vi "Clean Data.vi"(0 "Display State In":T1, 9 "Container State":T3, 11 "error in (no error)":errorcluster) -> (4 "Display State Out":T1, 15 "error out":errorcluster)   [LabVIEW 2017, in "3D Stem.xctl"]
uses:
  <vilib>/Math Plots/3D Math Plots/3D Stem/3D Stem XCtrl/3D Stem.xctl
  <vilib>/_xctls/Container State.ctl
  <vilib>/Math Plots/3D Math Plots/3D Stem/3D Stem XCtrl/State.ctl
  <vilib>/Math Plots/3D Math Plots/3D Stem/3D Stem/3D Stem.lvclass
  <vilib>/Math Plots/3D Math Plots/3D Plot/Action String/3DMathPlot Ctrl Act Queue.ctl
  <vilib>/Math Plots/3D Math Plots/3D Plot/Action String/3DMathPlot Ctrl Act Cluster.ctl
  <vilib>/Math Plots/3D Math Plots/3D Plot/Action String/3DMathPlot State Class.ctl
  <vilib>/_xctls/XControlSupport.lvlib
types:
  T1 = typedef "3D Stem.xctl/State.ctl" = cluster{"3D Stem.lvclass":refnum<class "3D Stem.lvclass">, "Control Ref Queue":T2, "Main Frame Color":u32, "Ramp Palette Color":u32, "Projection Palette Color":u32}
  T2 = typedef "3DMathPlot Ctrl Act Queue.ctl" = refnum<queue>
  T3 = typedef "XControlSupport.lvlib/Container State.ctl" = cluster{"Indicator?":bool, "Run Mode?":bool, " Refnum":refnum<vi>}
  T4 = typedef "3DMathPlot State Class.ctl" = enum16{"Update All Objects (Undo)", "Update Light Object Only", "Update Axis Object Only", "Update Plot Object Only", "Update Cursor Object Only", "Update Axis Plot Cursor Objects", "No Update"}
  T5 = typedef "3DMathPlot Ctrl Act Cluster.ctl" = cluster{"3D Picture Control":refnum<vi>, "Render Window Refnum":refnum<vi>, "XY Graph":refnum<vi>, "Intensity Graph":refnum<vi>, "Color Legend Palette":refnum<vi>, "Projection Palette":refnum<vi>, "XControl  Ref":refnum<vi>, "Facade Ref":refnum<vi>, "Export Image Ref":refnum<vi>, "Clear Data Flag":bool, "Display State Change Class":T4}
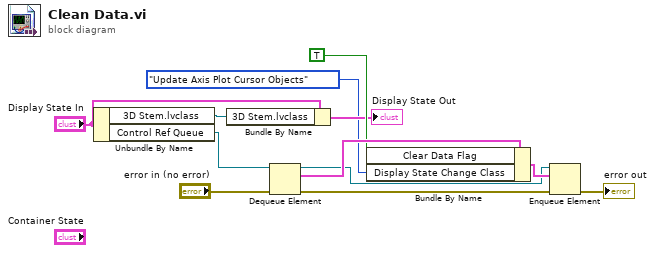
[diagram p0: block diagram]
diagram:
  n1 = Unbundle By Name("Display State In") -> ("3D Stem.lvclass"=w3:refnum<class "3D Stem.lvclass">, "Control Ref Queue"=w12:T2)
  n2 = Bundle By Name(cluster="Display State In", "3D Stem.lvclass"=w3) -> (→"Display State Out":T1)
  n3 = Dequeue Element(queue=w12, error in (no error)="error in (no error)") -> (queue out=w9:T2, element=w11:T5, error out=w7:errorcluster)  [unwired: 2 out]
  n4 = Bundle By Name(cluster=w11, "Clear Data Flag"=TRUE, "Display State Change Class"=3DMathPlot_State_Class."Update Axis Plot Cursor Objects") -> (w10:T5)
  n5 = Enqueue Element(queue=w9, element=w10, error in (no error)=w7) -> (error out=→"error out":errorcluster)  [unwired: 3 out]
